vi "getMirRotMat.vi"(7 "Num of Bending Mode":i32=20, 8 "error in (no error)":errorcluster, 9 "Skip Col Idx":i32[](array[numeric]), 10 "Mirror Subsystem":T1={"Mirror"="M1M3", "Actuatro Force File"="M1M3_1um_156_force.txt"}, 11 "BendModeToForce in":refnum<class "BendModeToForce.lvclass">) -> (0 "error out":errorcluster, 2 "Rotation Matrix":dbl[][](array[numeric]), 3 "BendModeToForce out":refnum<class "BendModeToForce.lvclass">)   [LabVIEW 2016, in "BendModeToForce.lvclass"]
doc: "Get the rotation matrix (row: actuator forces, col: bending modr) of specific mirror system."
uses:
  BendModeToForce.lvclass
  BendModeToForce.lvclass/BendModeToForce.ctl
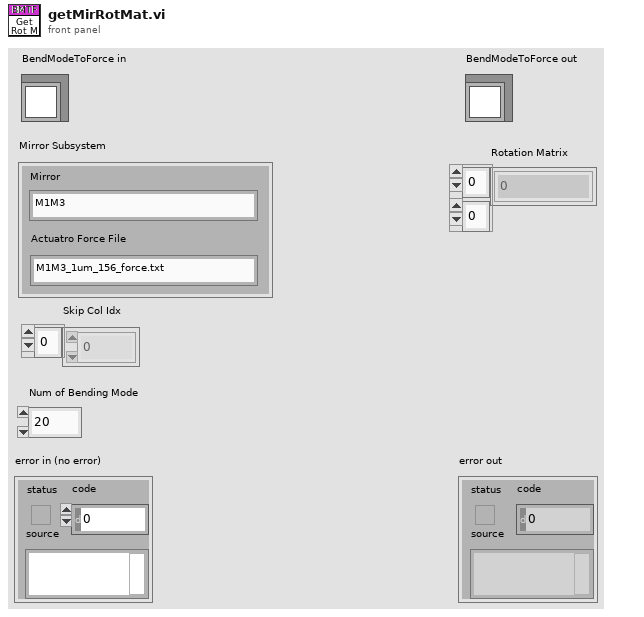
[diagram p1: front panel]
types:
  T1 = cluster{"Mirror":string, "Actuatro Force File":string}
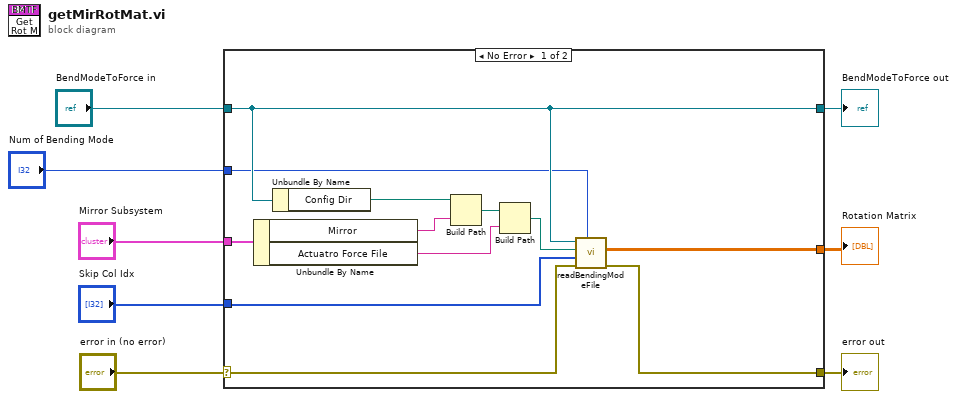
[diagram p0: block diagram]
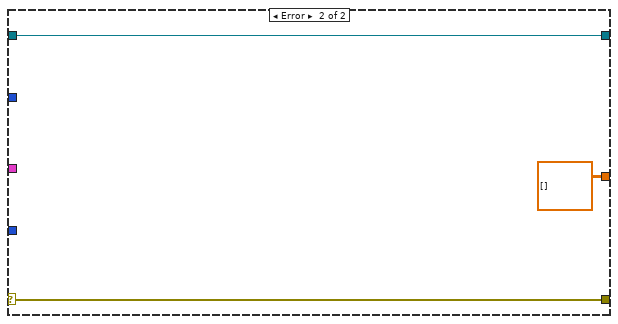
[diagram p2: hidden frame]
diagram:
  n1 = case shown="No Error" "error in (no error)" {
    selector: "error in (no error)" -> [w11 w23]
    tunnel: [w10 w23] -> w7
    tunnel: [w15 w22] -> w5
    tunnel: "BendModeToForce in" -> [w15 w22]
    tunnel: "Mirror Subsystem" -> [w20 _]
    tunnel: "Skip Col Idx" -> [w13 _]
    tunnel: "Num of Bending Mode" -> [w12 _]
    tunnel: [w9 dbl[][] [] ("Rotation Matrix")] -> w1
    frame No Error {
      n2 = Unbundle By Name(w20) -> ("Mirror"=w18:string, "Actuatro Force File"=w16:string)
      n3 = Unbundle By Name(w15) -> ("Config Dir"=w19:path)
      n4 = Build Path(base path=w19, name or relative path=w18) -> (appended path=w17:path)
      n5 = Build Path(base path=w17, name or relative path=w16) -> (appended path=w14:path)
      n6 = call "readBendingModeFile.vi"("Number of Bending Mode"=w12, "error in (no error)"=w11, "Skip Col Idx"=w13, "Path"=w14, "BendModeToForce in"=w15) -> ("error out"=w10:errorcluster, "Rotation Matrix"=w9:dbl[][])  [unwired: 4 in, 1 out]
    }
    frame Error {
    }
  }
  "error out" <- w7
  "BendModeToForce out" <- w5
  "Rotation Matrix" <- w1
